vi "Find Lines.vi"() -> ()   [LabVIEW 2011]
panel:
  out "Lines Calibrated (Shape Detection 1)":T1(array[cluster]) {"End Point"."Y" format="%.2f"; "End Point"."X" format="%.2f"; "Start Point"."Y" format="%.2f"; "Start Point"."X" format="%.2f"}
  out "Image Out":T2(plugin-control)
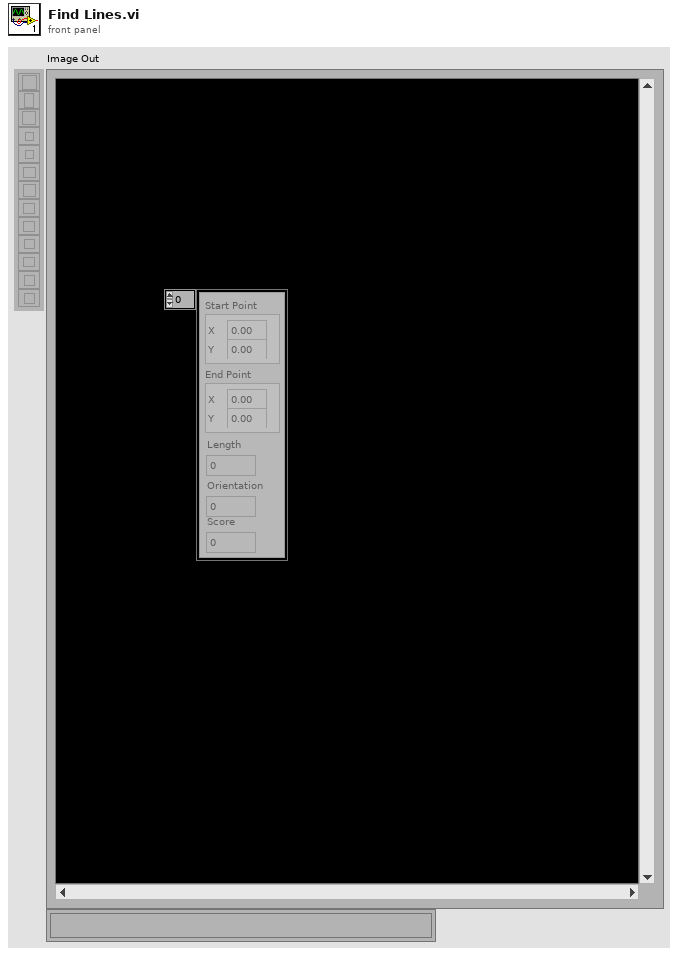
[diagram p1: front panel]
types:
  T1 = cluster{"Start Point":cluster{"X":sgl, "Y":sgl}, "End Point":cluster{"X":sgl, "Y":sgl}, "Length":dbl, "Orientation":dbl, "Score":dbl}[]
  T2 = typedef "IMAQ Image.ctl" = refnum<image>
  T3 = typedef "Image Type" = u32
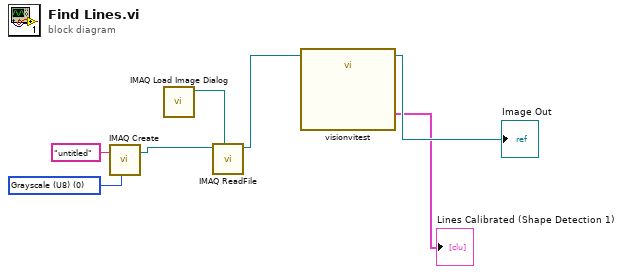
[diagram p0: block diagram]
diagram:
  w4 = T3 0 items=["Grayscale (U8)", "Grayscale (I16)", "Grayscale (SGL)", "Complex (CSG)", "RGB (U32)", "HSL (U32)", "RGB (U64)", "Grayscale (U16)"] ("Image Type")
  n1 = call "IMAQ Create"("Image Name"="untitled", "Image Type"=w4) -> ("New Image"=w7:T2)  [unwired: 3 in, 1 out]
  n2 = call "IMAQ Load Image Dialog"() -> ("Path"=w5:path)  [unwired: 9 in, 2 out]
  n3 = call "IMAQ ReadFile"("File Path"=w5, "Image"=w7) -> ("Image Out"=w3:T2)  [unwired: 5 in, 4 out]
  n4 = call "visionvitest.vi"("Image In"=w3) -> ("Image Out"=→"Image Out":T2, "Lines Calibrated (Shape Detection 1)"=→"Lines Calibrated (Shape Detection 1)":T1)  [unwired: 24 in, 1 out]
